vi "Receive Value Change Event.vi"(8 "error in (no error)":errorcluster, 10 "ValueChangeMsg":refnum<class "ValueChangeMsg.lvclass">, 11 "For Loop Dialog In":refnum<class "Subroutine Dialog.lvclass">) -> (0 "error out":errorcluster, 3 "For Loop Dialog Out":refnum<class "Subroutine Dialog.lvclass">)   [LabVIEW 2020, in "Subroutine Dialog.lvclass"]
doc: "<License>\nCopyright © 2017 Composed Systems, LLC | All rights reserved\nwww.composed.io\n\nAuthor: Ethan Stern <ethan.stern@composed.io>\n\nThis software is provided \"AS IS\" WITHOUT WARRANTIES, either express or implied, AND IS FOR EDUCATIONAL PURPOSES ONLY.\n</License>"
uses:
  <vilib>/gpm_packages/@cs/Test-executive-builder/Source/Test Executive Builder Dialogs/Edit Subroutine Dialog/Subroutine Dialog.lvclass
  C:/Program Files/National Instruments/LabVIEW 2020/vi.lib/ActorFramework/Actor/Actor.lvclass
  C:/Program Files/National Instruments/LabVIEW 2020/vi.lib/gpm_packages/@cs/popup-viewmanager/Source/Popup ViewManager/Popup ViewManager.lvclass
  C:/Program Files/National Instruments/LabVIEW 2020/vi.lib/gpm_packages/@cs/Test-executive-builder/Source/Test Executive Builder Dialogs/ITest Executive Builder Dialog/ITest Executive Builder Dialog.lvclass
  <vilib>/gpm_packages/@cs/mva-viewable/Source/ActorEvents/IEventAggregator Messages/ValueChangeMsg/ValueChangeMsg.lvclass
  <vilib>/gpm_packages/@cs/mva-viewable/Source/ActorEvents/IEventAggregator Messages/ValueChangeMsg/ValueChangeMsg.lvclass/ValueChangeMsg.ctl
  <vilib>/ActorFramework/Actor/Actor.lvclass/Actor.ctl
  <vilib>/ActorFramework/Message Enqueuer/Message Enqueuer.lvclass/Message Enqueuer.ctl
  <vilib>/gpm_packages/@cs/Test-executive-builder/Source/Test Executive Builder Dialogs/Edit Subroutine Dialog/Subroutine Dialog.lvclass/Subroutine Dialog.ctl
  <vilib>/gpm_packages/@cs/mva-viewable/Source/IViewable/IViewable Messages/Insert Front Panel Msg/Insert Front Panel Msg.lvclass/Insert Front Panel Msg.ctl
  <vilib>/gpm_packages/@cs/Test-executive-builder/Source/Test Executive Builder Dialogs/IAttribute Data Type View Messages/Set Value Msg/Set Value Msg.lvclass/Set Value Msg.ctl
  <vilib>/gpm_packages/@cs/Test-executive-builder/Source/Test Executive Builder Dialogs/ITest Executive Builder Dialog/ITest Executive Builder Dialog.lvclass/ITest Executive Builder Dialog.ctl
  87b0e31f-3c80-4f2a-a586-cd84fbbf9f86.vi
  5b375a54-e7cb-4e9e-8ad6-1d6d19e317aa.vi
  <vilib>/ActorFramework/Message Enqueuer/Init from Existing Queue.vi
  <vilib>/ActorFramework/Message Enqueuer/Enqueue.vi
  <vilib>/gpm_packages/@cs/Test-executive-builder/Source/Test Executive Builder Dialogs/ITest Executive Builder Dialog/Read Test Executive Ref.vi
  <vilib>/gpm_packages/@cs/Test-executive-builder/Source/Test Executive Builder Dialogs/ITest Executive Builder Dialog/Read GUID.vi
  <vilib>/gpm_packages/@cs/Test-executive-builder/Source/Test Executive Builder Dialogs/ITest Executive Builder Dialog/Read Data Type Handler Type.vi
  <vilib>/ActorFramework/Stop Msg/Stop Msg.lvclass
  C:/Program Files/National Instruments/LabVIEW 2020/vi.lib/ActorFramework/Message/Message.lvclass
  <vilib>/gpm_packages/@cs/mva-viewable/Source/IViewable/IViewable Messages/Insert Front Panel Msg/Insert Front Panel Msg.lvclass
  <vilib>/gpm_packages/@cs/Test-executive-builder/Source/Test Executive Builder Dialogs/IAttribute Data Type View Messages/Set Value Msg/Set Value Msg.lvclass
  <vilib>/ActorFramework/Message Priority Queue/Priority Enqueue.vi
  <vilib>/gpm_packages/@cs/test-executive/Source/Test Executive/TestExecutive Ref/Get Name.vi
  <vilib>/ActorFramework/Message Enqueuer/Message Enqueuer.lvclass
  <vilib>/gpm_packages/@cs/Test-executive-builder/Source/Test Executive Builder Dialogs/ITest Executive Builder Dialog/ITest Executive Builder Dialog.lvclass
  <vilib>/gpm_packages/@cs/Test-executive-builder/Source/Data Type Handler/Test Executive Builder Data Type Handler.lvclass
  <vilib>/ActorFramework/Actor/Actor.lvclass
  <vilib>/gpm_packages/@cs/popup-viewmanager/Source/Popup ViewManager/Popup ViewManager.lvclass
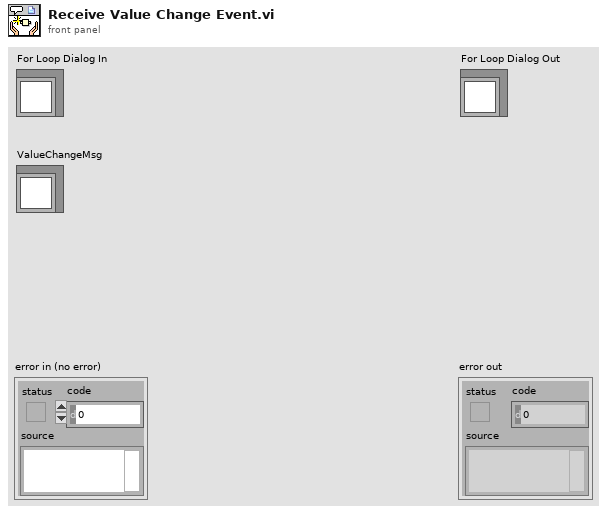
[diagram p1: front panel]
types:
  T1 = typedef "IViewable.lvlib/ProtectedSubpanel.lvclass/Protected Subpanel Reference.ctl" = refnum<data-value>
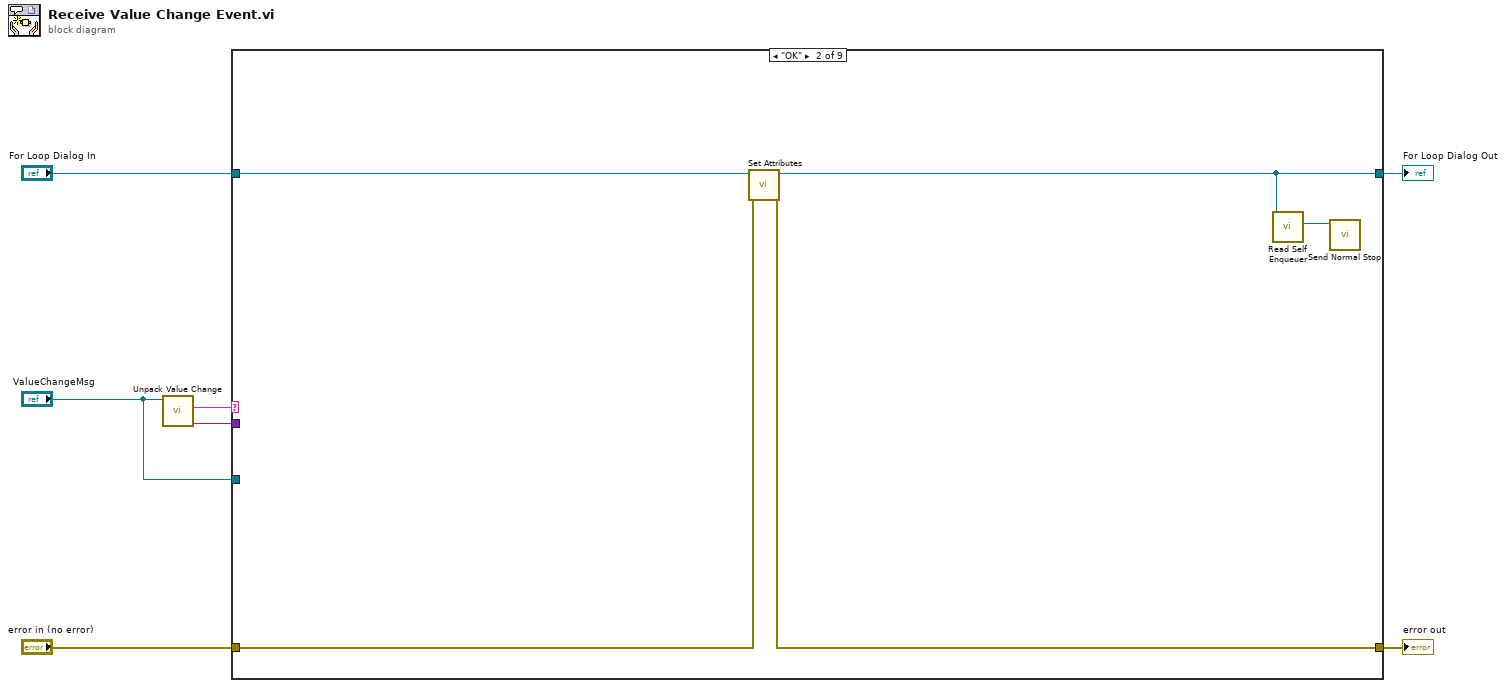
[diagram p0: block diagram]
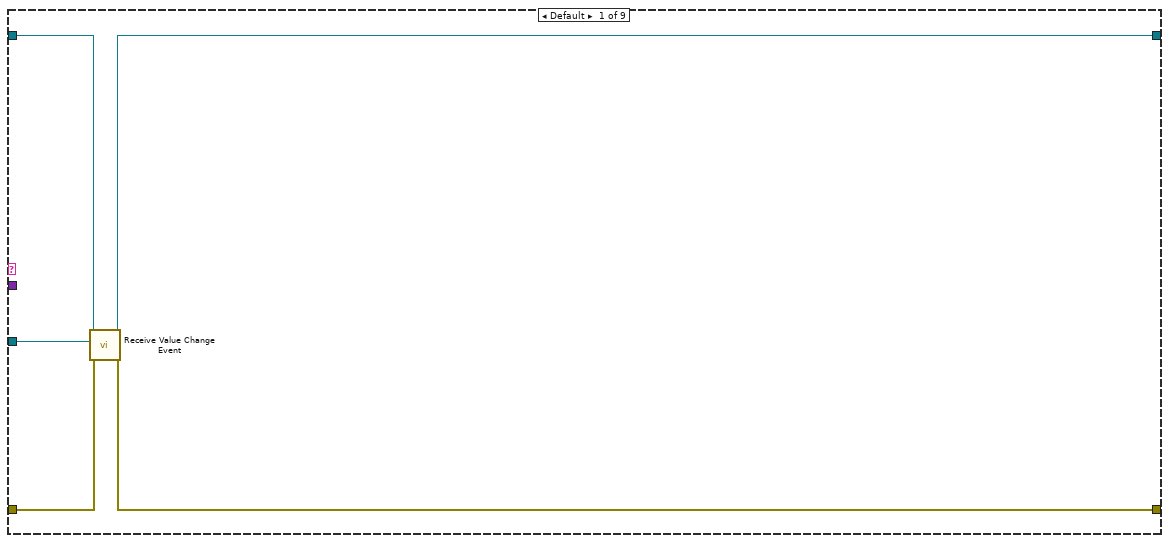
[diagram p2: hidden frame]
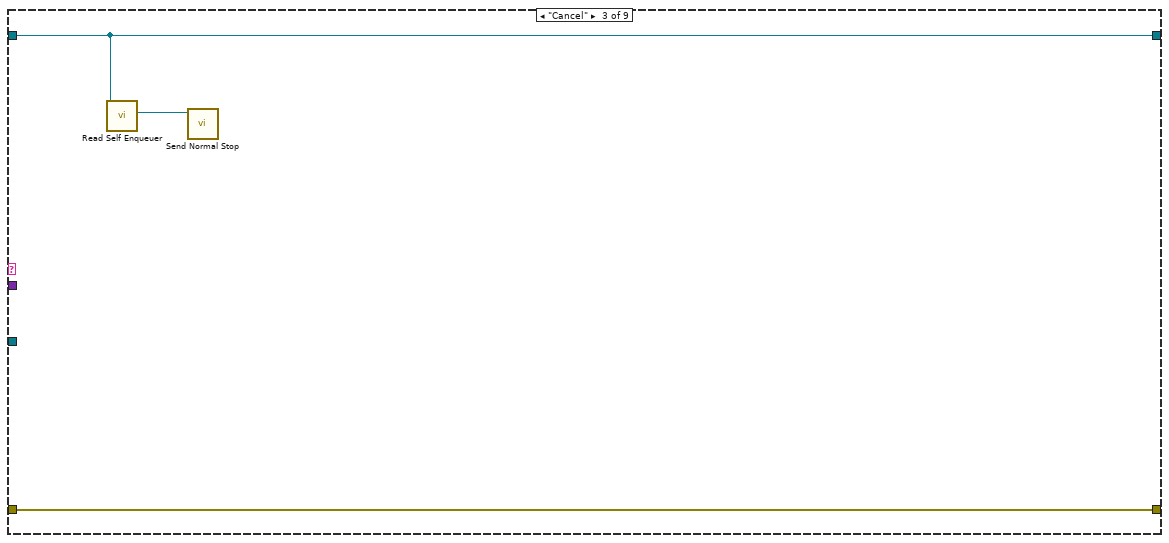
[diagram p3: hidden frame]
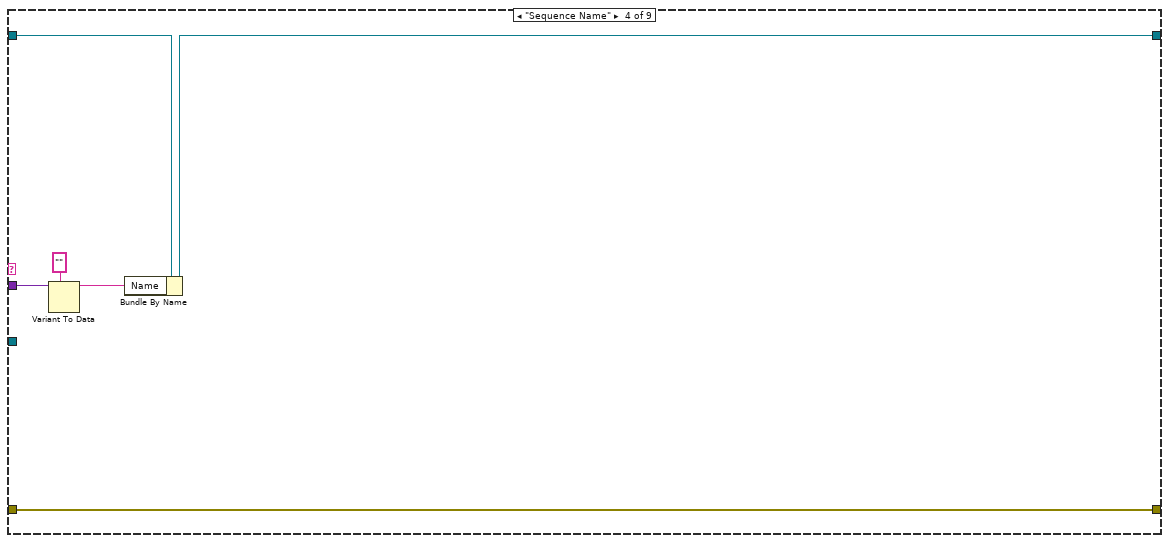
[diagram p4: hidden frame]
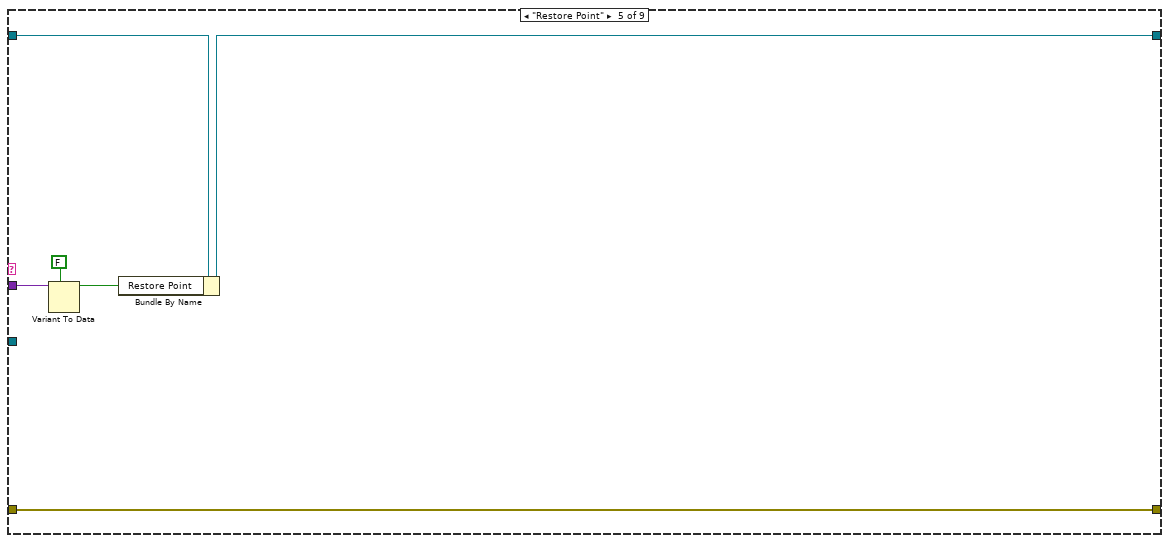
[diagram p5: hidden frame]
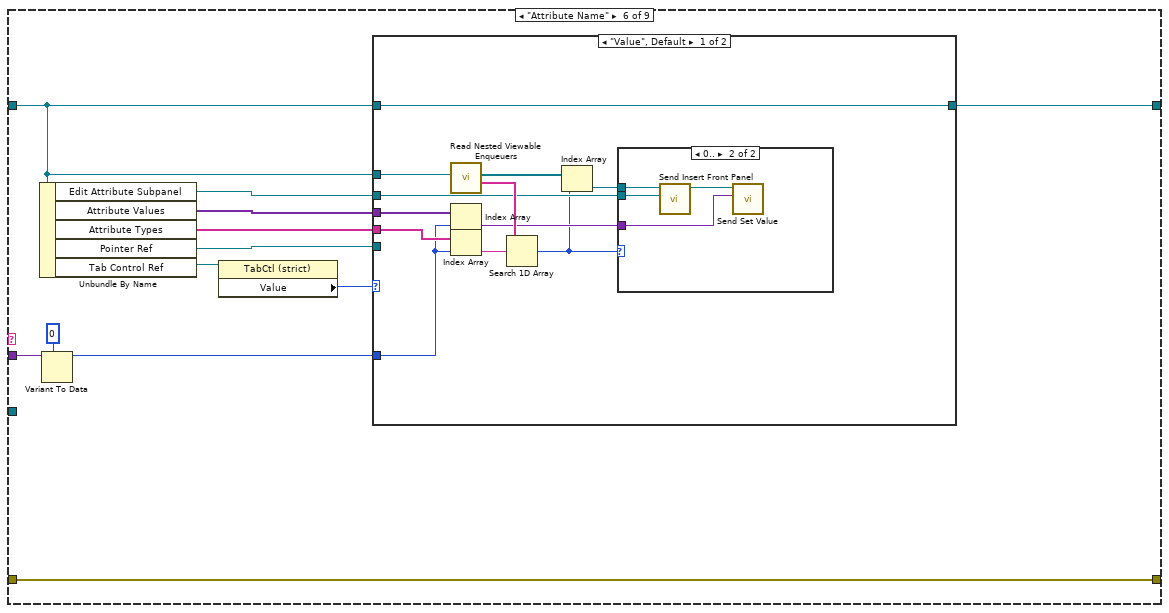
[diagram p6: hidden frame]
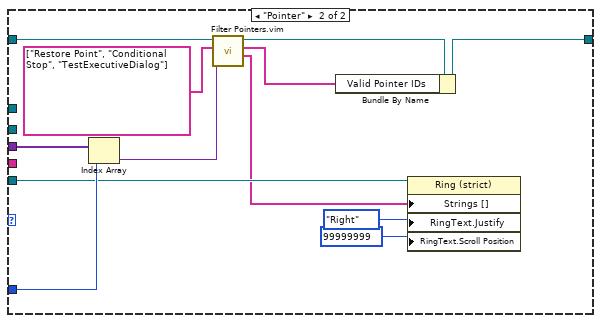
[diagram p8: hidden frame]
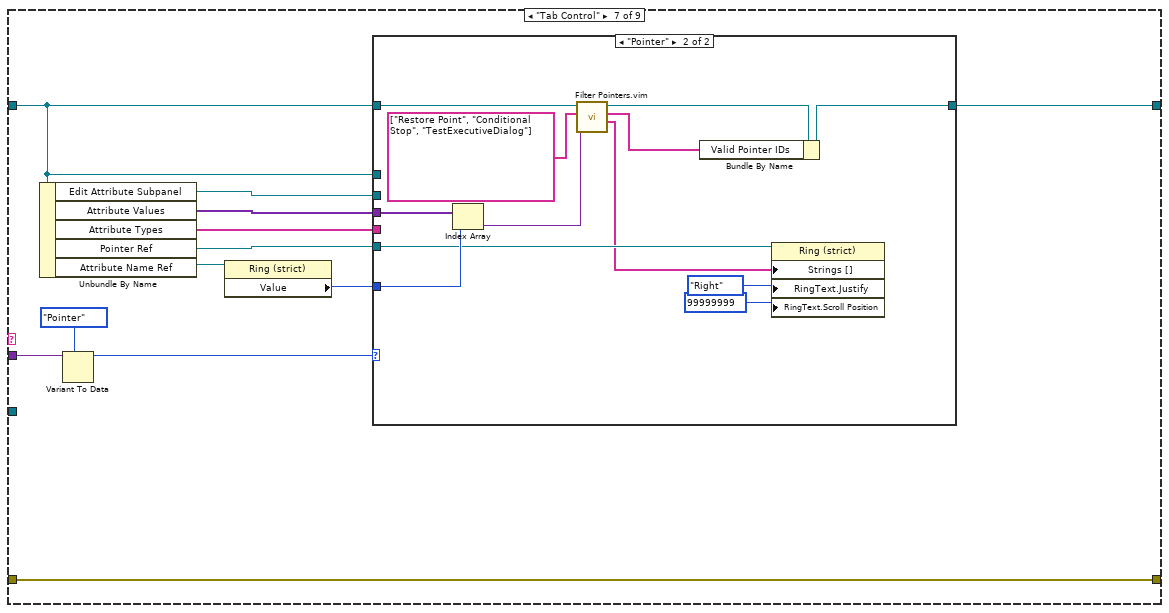
[diagram p9: hidden frame]
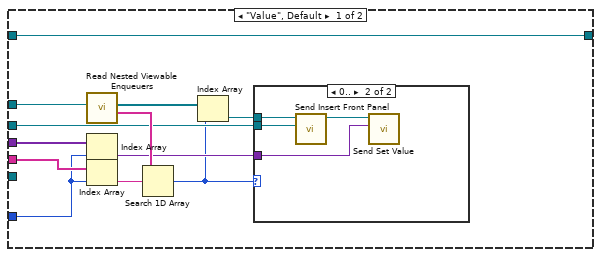
[diagram p10: hidden frame]
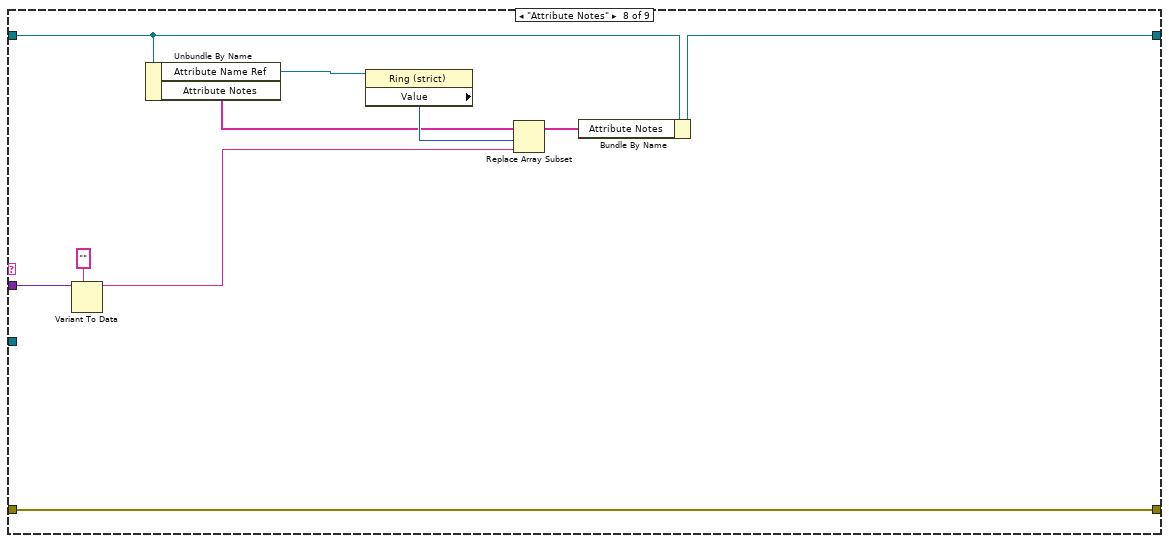
[diagram p12: hidden frame]
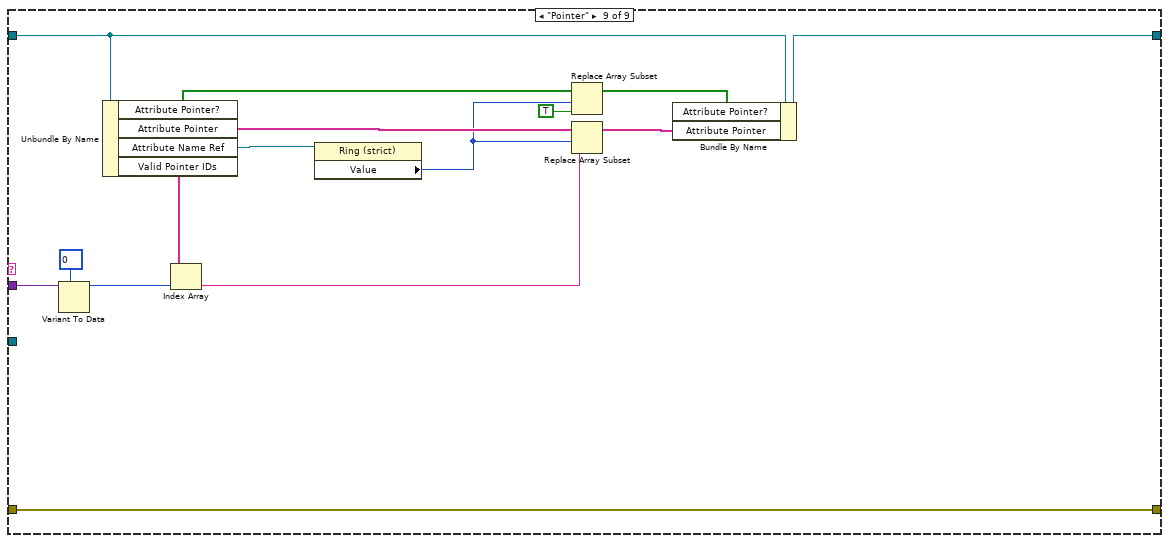
[diagram p13: hidden frame]
diagram:
  n1 = call <vilib>:"Unpack Value Change.vi"("ValueChangeMsg"="ValueChangeMsg") -> ("New Value"=w1:variant, "Control Label"=w2:string)  [unwired: 6 in, 3 out]
  n2 = case shown="\"OK\"" w2 {
    tunnel: [w12 w13 w20 w26 w32 w44 w84 w122 w137] -> w7
    tunnel: [w11 w15 w19 w21 w27 w35 w77 w114 w126] -> w6
    tunnel: "error in (no error)" -> [w10 w14 w20 w26 w32 w44 w84 w122 w137]
    tunnel: "For Loop Dialog In" -> [w9 w16 w19 w22 w28 w36 w78 w115 w127]
    tunnel: "ValueChangeMsg" -> [w8 _ _ _ _ _ _ _ _]
    tunnel: w1 -> [_ _ _ w25 w31 w43 w83 w118 w136]
    frame Default {
      n3 = call-parent "Receive Value Change Event.vi"("error in (no error)"=w10, "ValueChangeMsg"=w8, "IViewable In"=w9) -> ("error out"=w12:errorcluster, "IViewable Out"=w11:refnum<class "Subroutine Dialog.lvclass">)  [unwired: 7 in]
    }
    frame "OK" {
      n4 = call-dynamic "Set Attributes.vi"("error in (no error)"=w14, "Subroutine Dialog in"=w16) -> ("error out"=w13:errorcluster, "Subroutine Dialog out"=w15:refnum<class "Subroutine Dialog.lvclass">)  [unwired: 8 in]
      n5 = call <vilib>:"Read Self Enqueuer.vi"("Actor"=w15) -> ("Self Enqueuer"=w17:refnum<class "Message Enqueuer.lvclass">)  [unwired: 10 in]
      n6 = call <vilib>:"Send Normal Stop.vi"("Message Enqueuer"=w17) -> ()  [unwired: 10 in, 1 out]
    }
    frame "Cancel" {
      n7 = call <vilib>:"Read Self Enqueuer.vi"("Actor"=w19) -> ("Self Enqueuer"=w18:refnum<class "Message Enqueuer.lvclass">)  [unwired: 10 in]
      n8 = call <vilib>:"Send Normal Stop.vi"("Message Enqueuer"=w18) -> ()  [unwired: 10 in, 1 out]
    }
    frame "Sequence Name" {
      n9 = Variant To Data(type="" ("Iterations"), Variant=w25) -> (data=w23:string)  [unwired: 1 in, 1 out]
      n10 = Bundle By Name(cluster=w22, "Name"=w23) -> (w21:refnum<class "Subroutine Dialog.lvclass">)
    }
    frame "Restore Point" {
      n11 = Variant To Data(type=FALSE, Variant=w31) -> (data=w29:bool)  [unwired: 1 in, 1 out]
      n12 = Bundle By Name(cluster=w28, "Restore Point"=w29) -> (w27:refnum<class "Subroutine Dialog.lvclass">)
    }
    frame "Attribute Name" {
      n13 = Unbundle By Name(w36) -> ("Edit Attribute Subpanel"=w39:T1, "Attribute Values"=w40:variant[], "Attribute Types"=w41:string[], "Pointer Ref"=w33:refnum<vi>, "Tab Control Ref"=w37:refnum<vi>)
      n14 = Variant To Data(type=u16 0, Variant=w43) -> (data=w38:u16)  [unwired: 1 in, 1 out]
      n15 = property class="TabCtl (strict)"(reference=w37) -> ("Value"=w34:enum32{"Value", "Pointer"})  [unwired: 1 in, 2 out]
      n16 = case shown="\"Value\", Default" w34 {
        tunnel: w41 -> [w56 _]
        tunnel: w40 -> [w55 w71]
        tunnel: w39 -> [w50 _]
        tunnel: w36 -> [w48 _]
        tunnel: w38 -> [w47 w70]
        tunnel: [w45 w64] -> w35
        tunnel: w36 -> [w45 w72]
        tunnel: w33 -> [_ w67]
        frame "Value", Default {
          n17 = call <vilib>:"Read Nested Viewable Enqueuers.vi"("Popup ViewManager in"=w48) -> ("Viewable Names"=w52:string[], "Nested Enqueuers"=w54:refnum<class "Message Enqueuer.lvclass">[])  [unwired: 9 in]
          n18 = Index Array(array=w55, index=w47) -> (element=w49:variant)
          n19 = Index Array(array=w56, index=w47) -> (element=w51:string)
          n20 = Search 1D Array(1D array=w52, element=w51) -> (index of element=w46:i32)  [unwired: 1 in]
          n21 = Index Array(array=w54, index=w46) -> (element=w53:refnum<class "Message Enqueuer.lvclass">)
          n22 = case shown="0.." w46 {
            tunnel: w53 -> [_ w60]
            tunnel: w50 -> [_ w59]
            tunnel: w49 -> [_ w57]
            frame Default {
            }
            frame 0.. {
              n23 = call <vilib>:"Send Insert Front Panel.vi"("Protected Subpanel"=w59, "Message Enqueuer"=w60) -> ("Message Enqueuer out"=w58:refnum<class "Message Enqueuer.lvclass">)  [unwired: 8 in, 1 out]
              n24 = call <vilib>:"Send Set Value.vi"("Value"=w57, "Message Enqueuer"=w58) -> ()  [unwired: 8 in, 2 out]
            }
          }
        }
        frame "Pointer" {
          n25 = Index Array(array=w71, index=w70) -> (element=w69:variant)
          n26 = call "Filter Pointers.vim"("Type"=w69, "Exclusion List"=string[] ["Restore Point", "Conditional Stop", "TestExecutiveDialog"], "ITest Executive Builder Dialog in"=w72) -> ("Valid Pointer Names"=w66:string[], "Valid Pointer IDs"=w63:string[], "ITest Executive Builder Dialog out"=w65:refnum<class "Subroutine Dialog.lvclass">)  [unwired: 5 in, 1 out]
          n27 = Bundle By Name(cluster=w65, "Valid Pointer IDs"=w63) -> (w64:refnum<class "Subroutine Dialog.lvclass">)
          n28 = property class="Ring (strict)"(reference=w67, "Strings []"=w66, "RingText.Justify"=enum16{"Left", "Center", "Right"}."Right" ("Ring Text.Justification"), "RingText.Scroll Position"=u32 99999999 ("Ring Text.Scroll Position")) -> ()  [unwired: 1 in, 2 out]
        }
      }
    }
    frame "Tab Control" {
      n29 = Unbundle By Name(w78) -> ("Edit Attribute Subpanel"=w80:T1, "Attribute Values"=w81:variant[], "Attribute Types"=w82:string[], "Pointer Ref"=w76:refnum<vi>, "Attribute Name Ref"=w79:refnum<vi>)
      n30 = Variant To Data(type=enum32{"Value", "Pointer"}."Pointer" ("Tab Control"), Variant=w83) -> (data=w73:enum32{"Value", "Pointer"})  [unwired: 1 in, 1 out]
      n31 = property class="Ring (strict)"(reference=w79) -> ("Value"=w75:u16)  [unwired: 1 in, 2 out]
      n32 = case shown="\"Pointer\"" w73 {
        tunnel: w82 -> [w96 _]
        tunnel: w81 -> [w95 w111]
        tunnel: w80 -> [w90 _]
        tunnel: w78 -> [w88 _]
        tunnel: w75 -> [w87 w110]
        tunnel: [w85 w104] -> w77
        tunnel: w78 -> [w85 w112]
        tunnel: w76 -> [_ w107]
        frame "Value", Default {
          n33 = call <vilib>:"Read Nested Viewable Enqueuers.vi"("Popup ViewManager in"=w88) -> ("Viewable Names"=w92:string[], "Nested Enqueuers"=w94:refnum<class "Message Enqueuer.lvclass">[])  [unwired: 9 in]
          n34 = Index Array(array=w95, index=w87) -> (element=w89:variant)
          n35 = Index Array(array=w96, index=w87) -> (element=w91:string)
          n36 = Search 1D Array(1D array=w92, element=w91) -> (index of element=w86:i32)  [unwired: 1 in]
          n37 = Index Array(array=w94, index=w86) -> (element=w93:refnum<class "Message Enqueuer.lvclass">)
          n38 = case shown="0.." w86 {
            tunnel: w93 -> [_ w100]
            tunnel: w90 -> [_ w99]
            tunnel: w89 -> [_ w97]
            frame Default {
            }
            frame 0.. {
              n39 = call <vilib>:"Send Insert Front Panel.vi"("Protected Subpanel"=w99, "Message Enqueuer"=w100) -> ("Message Enqueuer out"=w98:refnum<class "Message Enqueuer.lvclass">)  [unwired: 8 in, 1 out]
              n40 = call <vilib>:"Send Set Value.vi"("Value"=w97, "Message Enqueuer"=w98) -> ()  [unwired: 8 in, 2 out]
            }
          }
        }
        frame "Pointer" {
          n41 = Index Array(array=w111, index=w110) -> (element=w109:variant)
          n42 = call "Filter Pointers.vim"("Type"=w109, "Exclusion List"=string[] ["Restore Point", "Conditional Stop", "TestExecutiveDialog"], "ITest Executive Builder Dialog in"=w112) -> ("Valid Pointer Names"=w106:string[], "Valid Pointer IDs"=w103:string[], "ITest Executive Builder Dialog out"=w105:refnum<class "Subroutine Dialog.lvclass">)  [unwired: 5 in, 1 out]
          n43 = Bundle By Name(cluster=w105, "Valid Pointer IDs"=w103) -> (w104:refnum<class "Subroutine Dialog.lvclass">)
          n44 = property class="Ring (strict)"(reference=w107, "Strings []"=w106, "RingText.Justify"=enum16{"Left", "Center", "Right"}."Right" ("Ring Text.Justification"), "RingText.Scroll Position"=u32 99999999 ("Ring Text.Scroll Position")) -> ()  [unwired: 1 in, 2 out]
        }
      }
    }
    frame "Attribute Notes" {
      n45 = Variant To Data(type="", Variant=w118) -> (data=w116:string)  [unwired: 1 in, 1 out]
      n46 = Unbundle By Name(w115) -> ("Attribute Name Ref"=w121:refnum<vi>, "Attribute Notes"=w119:string[])
      n47 = property class="Ring (strict)"(reference=w121) -> ("Value"=w120:u16)  [unwired: 1 in, 2 out]
      n48 = Replace Array Subset(array=w119, new element=w116, index=w120) -> (w113:string[])
      n49 = Bundle By Name(cluster=w115, "Attribute Notes"=w113) -> (w114:refnum<class "Subroutine Dialog.lvclass">)
    }
    frame "Pointer" {
      w135 = u16 0 items=[""] ("Pointer")
      n50 = Variant To Data(type=w135, Variant=w136) -> (data=w125:u16)  [unwired: 1 in, 1 out]
      n51 = Unbundle By Name(w127) -> ("Attribute Pointer?"=w132:bool[], "Attribute Pointer"=w133:string[], "Attribute Name Ref"=w134:refnum<vi>, "Valid Pointer IDs"=w124:string[])
      n52 = Index Array(array=w124, index=w125) -> (element=w123:string)
      n53 = property class="Ring (strict)"(reference=w134) -> ("Value"=w131:u16)  [unwired: 1 in, 2 out]
      n54 = Replace Array Subset(array=w132, new element=TRUE ("new element/subarray"), index=w131) -> (w128:bool[])
      n55 = Replace Array Subset(array=w133, new element=w123, index=w131) -> (w129:string[])
      n56 = Bundle By Name(cluster=w127, "Attribute Pointer?"=w128, "Attribute Pointer"=w129) -> (w126:refnum<class "Subroutine Dialog.lvclass">)
    }
  }
  "error out" <- w7
  "For Loop Dialog Out" <- w6
